vi "SQLGetInfo.vi"(4 "error in (no error)":errorcluster, 7 "ConnectionHandle":i32) -> (0 "error out":errorcluster, 2 "Info":string, 3 "OutputHandle":i32)   [LabVIEW 2011]
doc: "Execute entièrement la requête spécifiée par le lien"
uses:
  Odbc32.dll
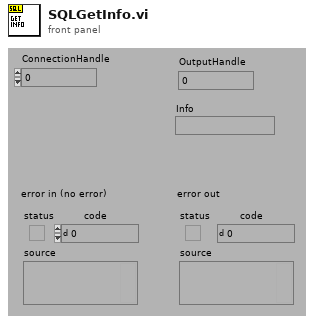
[diagram p1: front panel]
types:
  T1 = enum16{"NOPE", "SQL_HANDLE_ENV", "SQL_HANDLE_DBC", "SQL_HANDLE_STMT", "SQL_HANDLE_DESC"}
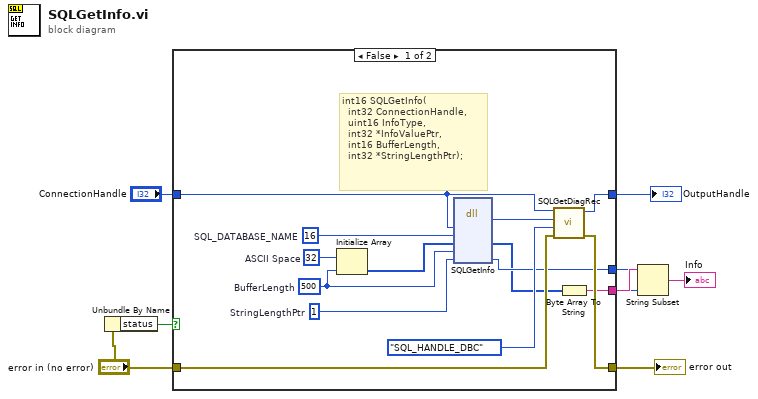
[diagram p0: block diagram]
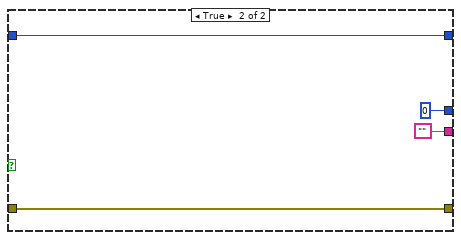
[diagram p2: hidden frame]
diagram:
  n1 = Unbundle By Name("error in (no error)") -> ("status"=w7:bool)
  n2 = case shown="False" w7 {
    tunnel: "ConnectionHandle" -> [w19 w25]
    tunnel: [w21 w26] -> w6
    tunnel: "error in (no error)" -> [w22 w26]
    tunnel: [w18 w25] -> w4
    tunnel: [w12 0 ("StringLengthPtr")] -> w1
    tunnel: [w9 ""] -> w3
    frame False {
      w15 = u8 32  # ASCII Space
      w14 = i16 500  # BufferLength
      w16 = u16 16  # SQL_DATABASE_NAME
      w13 = 1  # StringLengthPtr
      # "int16 SQLGetInfo(\n  int32 ConnectionHandle,\n  uint16 InfoType,\n  int32 *InfoValuePtr,\n  int16 BufferLength,\n  int32 *StringLengthPtr);"
      n3 = Initialize Array(w15, w14) -> (w11:u8[])
      n4 = dll-call lib="Odbc32.dll" fn="SQLGetInfo"("ConnectionHandle"=w19, "InfoType"=w16, "InfoValuePtr"=w11, "BufferLength"=w14, "StringLengthPtr"=w13) -> (w20:i16, "InfoValuePtr"=w10:u8[], "StringLengthPtr"=w12:i32)  [unwired: 6 in, 2 out]
      n5 = call "SQLGetDiagRec.vi"("error in (no error)"=w22, "HandleType"=T1."SQL_HANDLE_DBC", "Status (SQL_SUCCESS=0)"=w20, "Input Handle"=w19) -> ("error out"=w21:errorcluster, "Output Handle"=w18:i32)  [unwired: 2 out]
      n6 = Byte Array To String(unsigned byte array=w10) -> (string=w9:string)
    }
    frame True {
    }
  }
  "OutputHandle" <- w4
  "error out" <- w6
  n7 = String Subset(string=w3, length (rest)=w1) -> (substring=→"Info":string)  [unwired: 1 out]
